vi "Funktionen Schalten AutoKal.vi"() -> (3 "AutoKal":T1)   [LabVIEW 2020, in "Allgemein.lvlib"]
uses:
  Allgemein.lvlib
  FGV Analysator aktiv.ctl
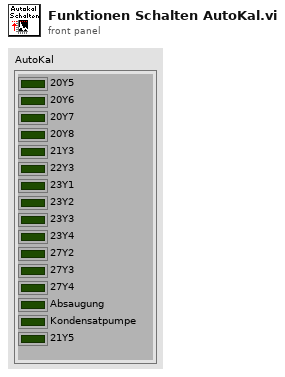
[diagram p1: front panel]
types:
  T1 = cluster{"20Y5":bool, "20Y6":bool, "20Y7":bool, "20Y8":bool, "21Y3":bool, "22Y3":bool, "23Y1":bool, "23Y2":bool, "23Y3":bool, "23Y4":bool, "27Y2":bool, "27Y3":bool, "27Y4":bool, "Absaugung":bool, "Kondensatpumpe":bool, "21Y5":bool}
  T2 = typedef "Allgemein.lvlib/FGV Analysator aktiv.ctl" = enum16{"lesen", "Analysator", "CG Aufschaltung", "KAL Zustand", "AutaKal GT?"}
  T3 = typedef "Auto Kalibrieren.lvlib/KalibrierZustaende.ctl" = cluster{"FTIR Zustand":u16, "PMA Zustand":u16, "FID CH4 Zustand":u16, "FID THC Zustand":u16, "FID THC CG":u16}
  T4 = typedef "Status Analysatoren.lvlib/Status Analysatoren_Anzeige.ctl" = cluster{"FT-IR":bool, "FID":bool, "PMA":bool}
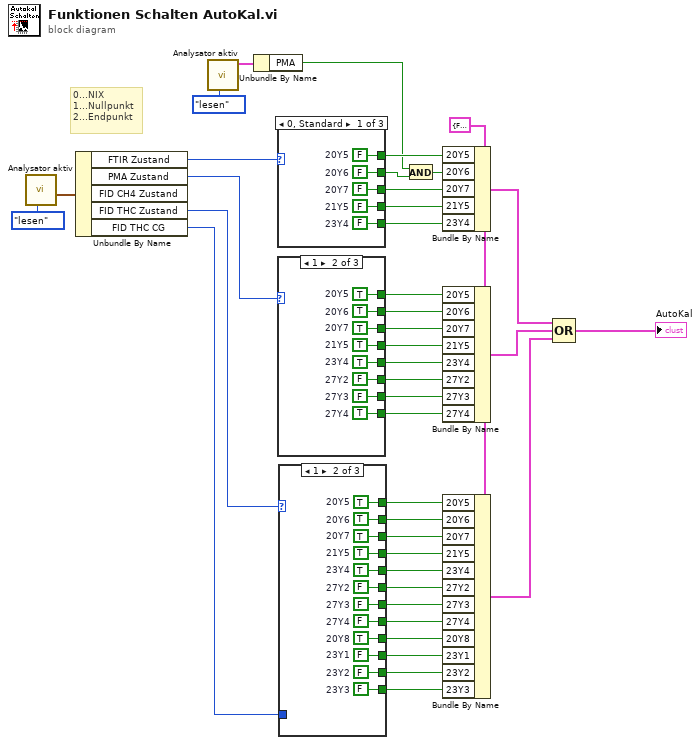
[diagram p0: block diagram]
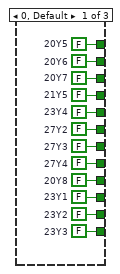
[diagram p2: hidden frame]
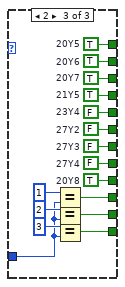
[diagram p3: hidden frame]
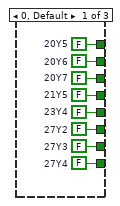
[diagram p4: hidden frame]
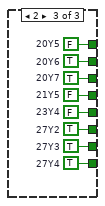
[diagram p5: hidden frame]
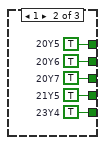
[diagram p6: hidden frame]
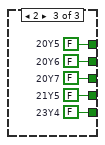
[diagram p7: hidden frame]
diagram:
  w5 = T1 {"20Y5"=FALSE, "20Y6"=FALSE, "20Y7"=FALSE, "20Y8"=FALSE, "21Y3"=FALSE, "22Y3"=FALSE, "23Y1"=FALSE, "23Y2"=FALSE, "23Y3"=FALSE, "23Y4"=FALSE, "27Y2"=FALSE, "27Y3"=FALSE, "27Y4"=FALSE, "Absaugung"=FALSE, "Kondensatpumpe"=FALSE, "21Y5"=FALSE} ("AutoKal")
  # "0...NIX\n1...Nullpunkt\n2...Endpunkt"
  n1 = call "Analysator aktiv.vi"("Aktion"=FGV_Analysator_aktiv."lesen") -> ("Kalibrieren"=w39:T3)  [unwired: 7 in, 3 out]
  n2 = Unbundle By Name(w39) -> ("FTIR Zustand"=w38:u16, "PMA Zustand"=w32:u16, "FID THC Zustand"=w23:u16, "FID THC CG"=w22:u16)  [unwired: 1 out]
  n3 = call "Analysator aktiv.vi"("Aktion"=FGV_Analysator_aktiv."lesen") -> ("Status Analysatoren"=w4:T4)  [unwired: 7 in, 3 out]
  n4 = Unbundle By Name(w4) -> ("PMA"=w1:bool)
  n5 = case shown="0, Standard" w38 {
    tunnel: [w45 w50 w55] -> w37
    tunnel: [w44 w49 w54] -> w35
    tunnel: [w42 w47 w52] -> w34
    tunnel: [w41 w46 w51] -> w33
    tunnel: [w43 w48 w53] -> w36
    frame 0, Default {
      w41 = FALSE  # 23Y4
      w42 = FALSE  # 21Y5
      w44 = FALSE  # 20Y7
      w43 = FALSE  # 20Y6
      w45 = FALSE  # 20Y5
    }
    frame 1 {
      w46 = TRUE  # 23Y4
      w47 = TRUE  # 21Y5
      w49 = TRUE  # 20Y7
      w48 = TRUE  # 20Y6
      w50 = TRUE  # 20Y5
    }
    frame 2 {
      w51 = FALSE  # 23Y4
      w52 = FALSE  # 21Y5
      w54 = FALSE  # 20Y7
      w53 = FALSE  # 20Y6
      w55 = FALSE  # 20Y5
    }
  }
  n6 = case shown="1" w32 {
    tunnel: [w63 w71 w79] -> w31
    tunnel: [w62 w70 w78] -> w29
    tunnel: [w60 w68 w76] -> w28
    tunnel: [w59 w67 w75] -> w27
    tunnel: [w58 w66 w74] -> w26
    tunnel: [w57 w65 w73] -> w25
    tunnel: [w56 w64 w72] -> w24
    tunnel: [w61 w69 w77] -> w30
    frame 0, Default {
      w56 = FALSE  # 27Y4
      w57 = FALSE  # 27Y3
      w58 = FALSE  # 27Y2
      w59 = FALSE  # 23Y4
      w60 = FALSE  # 21Y5
      w62 = FALSE  # 20Y7
      w61 = FALSE  # 20Y6
      w63 = FALSE  # 20Y5
    }
    frame 1 {
      w64 = TRUE  # 27Y4
      w65 = FALSE  # 27Y3
      w66 = FALSE  # 27Y2
      w67 = TRUE  # 23Y4
      w68 = TRUE  # 21Y5
      w70 = TRUE  # 20Y7
      w69 = TRUE  # 20Y6
      w71 = TRUE  # 20Y5
    }
    frame 2 {
      w72 = TRUE  # 27Y4
      w73 = TRUE  # 27Y3
      w74 = TRUE  # 27Y2
      w75 = FALSE  # 23Y4
      w76 = FALSE  # 21Y5
      w78 = TRUE  # 20Y7
      w77 = TRUE  # 20Y6
      w79 = FALSE  # 20Y5
    }
  }
  n7 = case shown="1" w23 {
    tunnel: [w91 w103 w119] -> w21
    tunnel: [w90 w102 w118] -> w19
    tunnel: [w88 w100 w116] -> w18
    tunnel: [w87 w99 w115] -> w17
    tunnel: [w86 w98 w114] -> w16
    tunnel: [w85 w97 w113] -> w15
    tunnel: [w84 w96 w112] -> w14
    tunnel: [w83 w95 w111] -> w13
    tunnel: [w89 w101 w117] -> w20
    tunnel: w22 -> [_ _ w104]
    tunnel: [w80 w92 w107] -> w12
    tunnel: [w81 w93 w106] -> w11
    tunnel: [w82 w94 w105] -> w10
    frame 0, Default {
      w82 = FALSE  # 23Y3
      w81 = FALSE  # 23Y2
      w80 = FALSE  # 23Y1
      w83 = FALSE  # 20Y8
      w84 = FALSE  # 27Y4
      w85 = FALSE  # 27Y3
      w86 = FALSE  # 27Y2
      w87 = FALSE  # 23Y4
      w88 = FALSE  # 21Y5
      w90 = FALSE  # 20Y7
      w89 = FALSE  # 20Y6
      w91 = FALSE  # 20Y5
    }
    frame 1 {
      w94 = FALSE  # 23Y3
      w93 = FALSE  # 23Y2
      w92 = FALSE  # 23Y1
      w95 = TRUE  # 20Y8
      w96 = FALSE  # 27Y4
      w97 = FALSE  # 27Y3
      w98 = FALSE  # 27Y2
      w99 = TRUE  # 23Y4
      w100 = TRUE  # 21Y5
      w102 = TRUE  # 20Y7
      w101 = TRUE  # 20Y6
      w103 = TRUE  # 20Y5
    }
    frame 2 {
      w111 = TRUE  # 20Y8
      w112 = FALSE  # 27Y4
      w113 = FALSE  # 27Y3
      w114 = FALSE  # 27Y2
      w115 = FALSE  # 23Y4
      w116 = TRUE  # 21Y5
      w118 = TRUE  # 20Y7
      w117 = TRUE  # 20Y6
      w119 = TRUE  # 20Y5
      n8 = Equal?(x=u16 1, y=w104) -> (x = y?=w107:bool)
      n9 = Equal?(x=u16 2, y=w104) -> (x = y?=w106:bool)
      n10 = Equal?(x=u16 3, y=w104) -> (x = y?=w105:bool)
    }
  }
  n11 = And(x=w1, y=w36) -> (x .and. y?=w2:bool)
  n12 = Bundle By Name(cluster=w5, "20Y5"=w37, "20Y6"=w2, "20Y7"=w35, "21Y5"=w34, "23Y4"=w33) -> (w9:T1)
  n13 = Bundle By Name(cluster=w5, "20Y5"=w31, "20Y6"=w30, "20Y7"=w29, "21Y5"=w28, "23Y4"=w27, "27Y2"=w26, "27Y3"=w25, "27Y4"=w24) -> (w8:T1)
  n14 = Bundle By Name(cluster=w5, "20Y5"=w21, "20Y6"=w20, "20Y7"=w19, "21Y5"=w18, "23Y4"=w17, "27Y2"=w16, "27Y3"=w15, "27Y4"=w14, "20Y8"=w13, "23Y1"=w12, "23Y2"=w11, "23Y3"=w10) -> (w7:T1)
  n15 = Compound Arithmetic op=OR ("Mehrfacharithmetik")(w9, w8, w7) -> (→"AutoKal":T1)
